vi "GetSet Handle.vi"(7 "store (F)":bool, 8 "error in":errorcluster, 9 "handle in":u64, 10 "connection":string, 11 "LINX Base in":refnum<class "LINX Base.lvclass">) -> (0 "error out":errorcluster, 1 "handle out":u64, 2 "name":string, 3 "LINX Base out":refnum<class "LINX Base.lvclass">)   [LabVIEW 2020, in "LINX Base.lvclass"]
uses:
  LINX Base.lvclass
  LINX Base.lvclass/LINX Base.ctl
  Typedef/Error Type.ctl
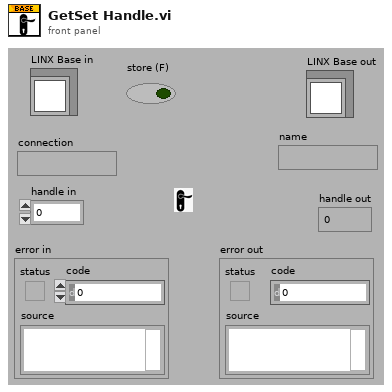
[diagram p1: front panel]
types:
  T1 = typedef "LINX Base.lvclass/Error Type.ctl" = enum16{"Unknown", "Timeout", "Corrupt Return Packet", "Unable To Connect", "Command Not Supported", "Channel DNE", "Invalid COM Config", "Firmware Version Mismatch", "myRIO Support", "CMD Specific Error", "Local IO Not Supported"}
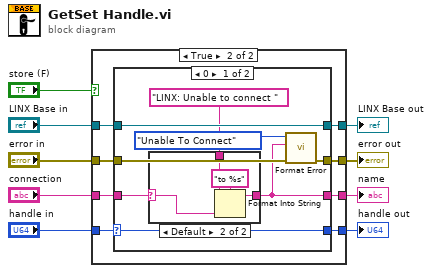
[diagram p0: block diagram]
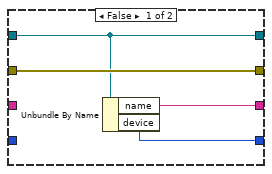
[diagram p2: hidden frame]
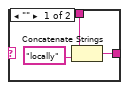
[diagram p3: hidden frame]
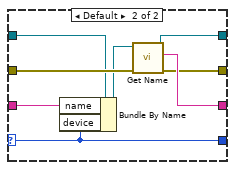
[diagram p4: hidden frame]
diagram:
  n1 = case shown="True" "store (F)" {
    tunnel: "LINX Base in" -> [w12 w21]
    tunnel: [w12 w20] -> w8
    tunnel: [w13 w19] -> w7
    tunnel: [w11 w18] -> w6
    tunnel: "handle in" -> [_ w17]
    tunnel: "error in" -> [w13 w16]
    tunnel: "connection" -> [_ w15]
    tunnel: [w10 w14] -> w1
    frame False {
      n2 = Unbundle By Name(w12) -> ("name"=w11:string, "device"=w10:u64)
    }
    frame True {
      n3 = case shown="0" w17 {
        selector: w17 -> [w25 w37]
        tunnel: [w22 w44] -> w18
        tunnel: [w27 w43] -> w19
        tunnel: w16 -> [w28 w42]
        tunnel: [w29 w41] -> w20
        tunnel: w21 -> [w29 w40]
        tunnel: w15 -> [w24 w38]
        tunnel: [w25 w37] -> w14
        frame 0 {
          n4 = case shown="Default" w24 {
            selector: w24 -> [_ w36]
            tunnel: "LINX: Unable to connect " ("format string") -> [w31 w35]
            tunnel: [w32 w34] -> w22
            frame "" {
              n5 = Concatenate Strings(w31, "locally") -> (w32:string)
            }
            frame Default {
              n6 = Format Into String(format string="to %s", initial string=w35, w36) -> (resulting string=w34:string)  [unwired: 1 in, 1 out]
            }
          }
          n7 = call "Format Error.vi"("error in (no error)"=w28, "Message"=w22, "Error Type"=Error_Type."Unable To Connect") -> ("error out"=w27:errorcluster)  [unwired: 8 out]
        }
        frame Default {
          n8 = Bundle By Name(cluster=w40, "name"=w38, "device"=w37) -> (w39:refnum<class "LINX Base.lvclass">)
          n9 = call "Get Name.vi"("error in (no error)"=w42, "LINX Base in"=w39) -> ("error out"=w43:errorcluster, "name"=w44:string, "LINX Base out"=w41:refnum<class "LINX Base.lvclass">)  [unwired: 7 out]
        }
      }
    }
  }
  "LINX Base out" <- w8
  "error out" <- w7
  "name" <- w6
  "handle out" <- w1
